vi "Initbrd_SD.vi"(0 "AdrDelay":u32=4096 format="%.0x", 1 "burst":u8, 2 "sym":u8=1, 3 "waits":u32, 4 "pixel":u32=5400, 5 "flag816":u32=2) -> ()   [LabVIEW 2015]
uses:
  DLL/ESLSCDLL.dll
panel:
  in  "pclk":u32=2 format="%.0x"
  in  "PPortAddress":u32=888 format="%.0x"
  # "set read frequency"
  # "8bit=2/12-16bit=1"
  # "not used"
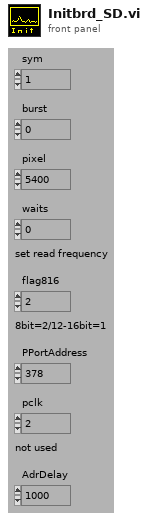
[diagram p1: front panel]
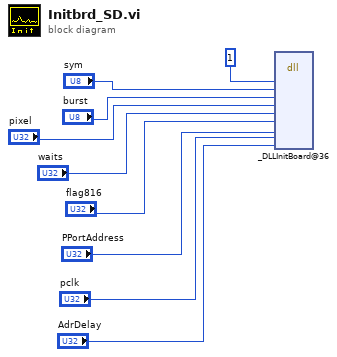
[diagram p0: block diagram]
diagram:
  n1 = dll-call lib="G:/SD/TRANCON/DLL/ESLSCDLL.dll" fn="_DLLInitBoard@36"("drv"=u32 1, "sym"="sym", "burst"="burst", "pixel"="pixel", "waits"="waits", "flag816"="flag816", "pportadr"="PPortAddress", "pclk"="pclk", "xckdelay"="AdrDelay") -> ()  [unwired: 13 in, 2 out]
